vi "读取-LH机械手-拍照位.vi"(5 "错误输入（无错误）":errorcluster, 9 "连接ID":refnum<k5>) -> (0 "y":dbl, 1 "x":dbl, 2 "Arrived":bool, 3 "连接ID 2":refnum<k5>, 4 "error out":errorcluster)   [LabVIEW 2016]
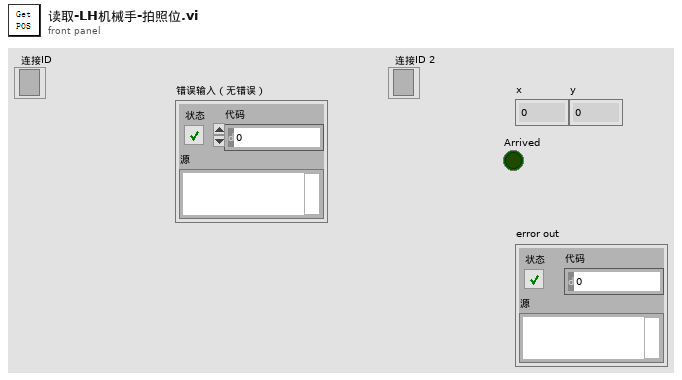
[diagram p1: front panel]
types:
  T1 = enum16{"Standard", "Buffered", "CRLF", "Immediate"}
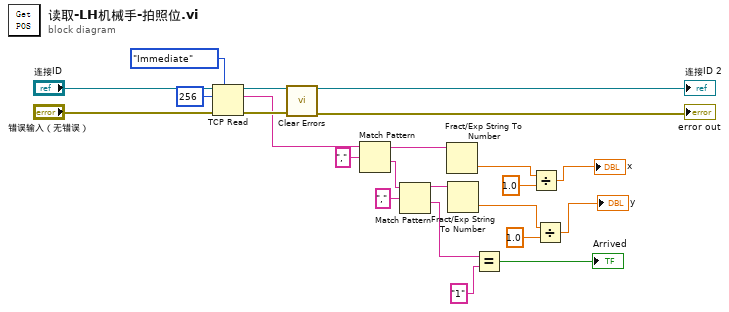
[diagram p0: block diagram]
diagram:
  n1 = TCP Read(connection ID="连接ID", bytes to read=256 ("读取的字节"), error in (no error)="错误输入（无错误）", 7:T1."Immediate" ("模式（标准）")) -> (connection ID out=→"连接ID 2":refnum<k5>, data out=w8:string, error out=w17:errorcluster)  [unwired: 1 in]
  n2 = call <vilib>:"Clear Errors.vi"("error in (no error)"=w17) -> ("error out"=→"error out":errorcluster)  [unwired: 5 in, 1 out]
  n3 = Match Pattern(string=w8, regular expression="," ("正则表达式")) -> (before substring=w20:string, after substring=w12:string)  [unwired: 1 in, 2 out]
  n4 = Match Pattern(string=w12, regular expression="," ("正则表达式")) -> (before substring=w11:string, after substring=w9:string)  [unwired: 1 in, 2 out]
  n5 = Fract/Exp String To Number(string=w20) -> (number=w5:dbl)  [unwired: 3 in, 1 out]
  n6 = Fract/Exp String To Number(string=w11) -> (number=w2:dbl)  [unwired: 3 in, 1 out]
  n7 = Equal?(x=w9, y="1" ("x")) -> (x = y?=→"Arrived":bool)
  n8 = Divide(x=w5, y=1.0) -> (x/y=→"x":dbl)
  n9 = Divide(x=w2, y=1.0) -> (x/y=→"y":dbl)
